vi "setUp.vi"(8 "error in (no error)":errorcluster, 11 "reference in":refnum<class "[Test Case] File or directory exists.lvclass">=refnum) -> (0 "error out":errorcluster, 3 "reference out":refnum<class "[Test Case] File or directory exists.lvclass">)   [LabVIEW 2016, in "Tests.lvlib" / "[Test Case] File or directory exists.lvclass"]
doc: "setUp runs prior to the test method during test execution. Use this method to initialize any object data required by your tests."
uses:
  [Test Case] File or directory exists.lvclass
  classes/File Transfer Behavior/File Transfer Behavior.lvclass
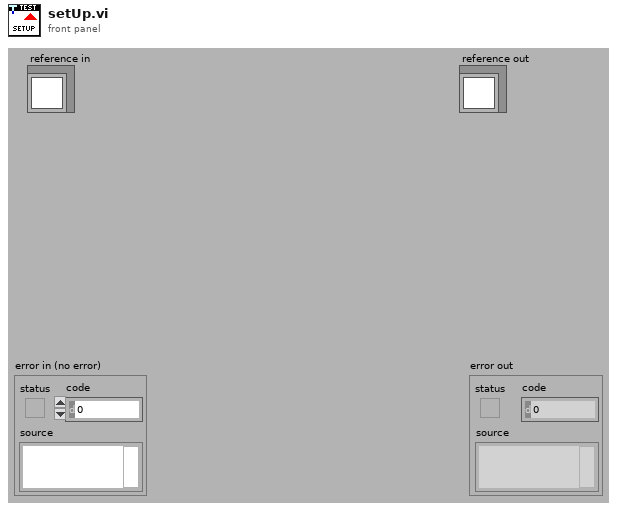
[diagram p1: front panel]
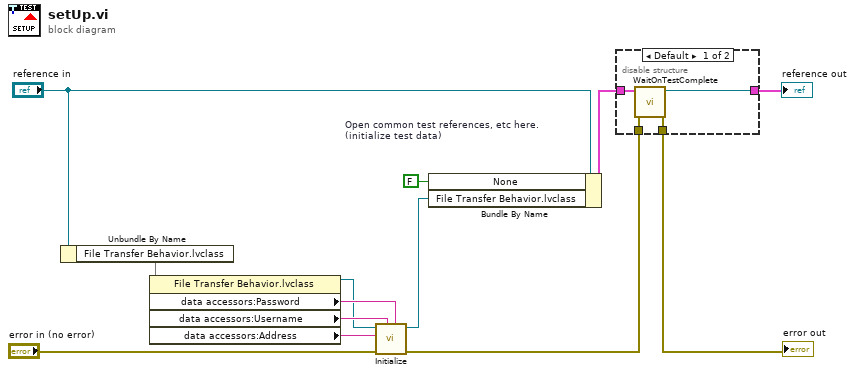
[diagram p0: block diagram]
diagram:
  w10 = FALSE  # Open common test references, etc here. (initialize test data)
  n1 = Unbundle By Name("reference in") -> ("File Transfer Behavior.lvclass"=w2)
  n2 = property class="File Transfer Behavior.lvclass"(reference=w2) -> (reference out=w1:refnum<class "File Transfer Behavior.lvclass">, "data accessors:Password"=w5:string, "data accessors:Username"=w4:string, "data accessors:Address"=w3:string)  [unwired: 1 in, 1 out]
  n3 = call-dynamic "Initialize.vi"("Password"=w5, "Username"=w4, "error in (no error)"="error in (no error)", "Address"=w3, "File Transfer Behavior in"=w1) -> ("error out"=w8:errorcluster, "File Transfer Behavior out"=w7:refnum<class "File Transfer Behavior.lvclass">)  [unwired: 5 in]
  n4 = Bundle By Name(cluster="reference in", "None"=w10, "File Transfer Behavior.lvclass"=w7) -> (w11:cluster{})
  n5 = disable-structure shown="Default" {
    disable-tunnel: w8 -> [w17 w18]
    disable-tunnel: [w16 w18] -> w13
    disable-tunnel: [w15 w19] -> w12
    disable-tunnel: w11 -> [w14 w19]
    frame condition #0 (active) {
      n6 = call <vilib>:"WaitOnTestComplete.vi"("error in (no error)"=w17, "TestCase in"=w14) -> ("error out"=w16:errorcluster, "TestCase out"=w15:refnum<class "[Test Case] File or directory exists.lvclass">)  [unwired: 8 in]
    }
    frame condition #1 {
    }
  }
  "error out" <- w13
  "reference out" <- w12
